vi "GetTestMap_AfterStartTest_ContainsOneElement.vi"() -> ()   [LabVIEW 2017, in "ResultTreeListener.Tests.lvlib"]
uses:
  ResultTreeListener.Tests.lvlib
  Support/FakeTestCase/FakeTestCase.lvclass
  C:/Users/de200256/Code/logmanoriginal/lvunit/Test/Test.lvclass
  ResultTreeListener/ResultTreeListener.lvclass
  ResultTree/ResultTree.lvclass
  Assertion/Assertion.lvlib
  Test/Test.lvclass
panel:
  out "error out":errorcluster
  in  "Tree":string(tree)
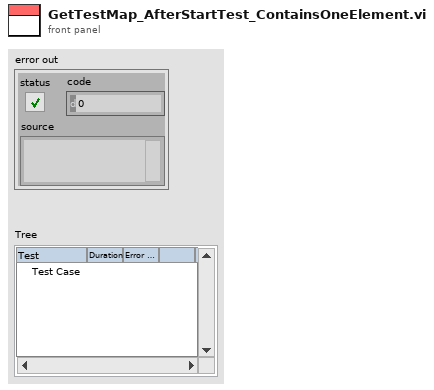
[diagram p1: front panel]
types:
  T1 = cluster{"Tag":string, "Test":refnum<class "Test.lvclass">}[]
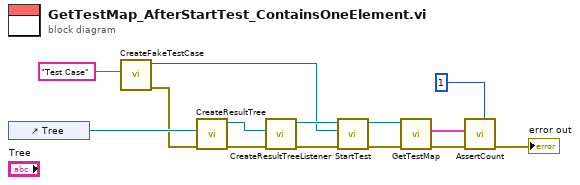
[diagram p0: block diagram]
diagram:
  n1 = control-ref of="Tree"() -> (w7:refnum<vi>)
  n2 = call "CreateFakeTestCase.vi"("Name"="Test Case") -> ("error out"=w5:errorcluster, "FakeTestCase out"=w9:refnum<class "FakeTestCase.lvclass">)  [unwired: 9 in]
  n3 = call "CreateResultTree.vi"("error in (no error)"=w5, "Tree Refnum"=w7) -> ("error out"=w14:errorcluster, "ResultTree out"=w13:refnum<class "ResultTree.lvclass">)  [unwired: 8 in]
  n4 = call "CreateResultTreeListener.vi"("error in (no error)"=w14, "ResultTree"=w13) -> ("error out"=w12:errorcluster, "ResultTreeListener out"=w10:refnum<class "ResultTreeListener.lvclass">)  [unwired: 8 in]
  n5 = call-dynamic "StartTest.vi"("error in (no error)"=w12, "Test"=w9, "ResultTreeListener in"=w10) -> ("error out"=w6:errorcluster, "ResultTreeListener out"=w2:refnum<class "ResultTreeListener.lvclass">)  [unwired: 7 in]
  n6 = call "GetTestMap.vi"("error in (no error)"=w6, "ResultTreeListener in"=w2) -> ("error out"=w3:errorcluster, "Test Map"=w1:T1)  [unwired: 7 in, 1 out]
  n7 = call "AssertCount.vi"("Expected"=1, "error in (no error)"=w3, "Haystack"=w1) -> ("error out"=→"error out":errorcluster)  [unwired: 8 in]
